vi "DragItem.vi"(8 "error in (no error)":errorcluster, 11 "OrderSelection in":refnum<class "OrderSelection.lvclass">) -> (0 "error out":errorcluster, 3 "OrderSelection out":refnum<class "OrderSelection.lvclass">)   [LabVIEW 2015, in "OrderSelection.lvclass"]
uses:
  OrderSelection.lvclass
  <vilib>/Utility/miscctls.llb/LVPointTypeDef.ctl
  OrderSelection.lvclass/OrderSelection.ctl
  Read ItemGraphic.vi
  Read Items.vi
  Read SelectedItem.vi
  <vilib>/Utility/inputDevices.llb/mouseAcquire.vi
  <vilib>/Utility/inputDevices.llb/closeMouse.vi
panel:
  out "SelectedItem":picture
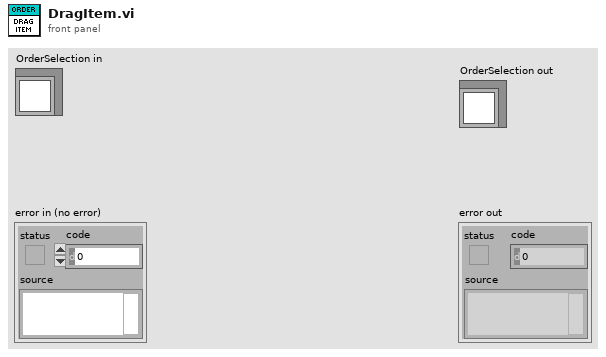
[diagram p1: front panel]
types:
  T1 = typedef "LVPointTypeDef.ctl" = cluster{"Horizontal":i16, "Vertical":i16}
  T2 = enum32{"Invalid", "Standard", "Closed", "Hidden", "Minimized", "Maximized"}
  T3 = cluster{"horizontal":enum16{"left", "center", "right"}, "vertical":enum16{"top", "center", "bottom"}}
  T4 = typedef "imagedata.ctl" = cluster{"image type":i32, "image depth":i32, "image":u8[], "mask":u8[], "colors":u32[], "Rectangle":cluster{"left":i16, "top":i16, "right":i16, "bottom":i16}}
  T5 = typedef "LVRectTypeDef.ctl" = cluster{"Left":i16, "Top":i16, "Right":i16, "Bottom":i16}
  T6 = cluster{"Horizontal":i32, "Vertical":i32, "Scrolling":i32}
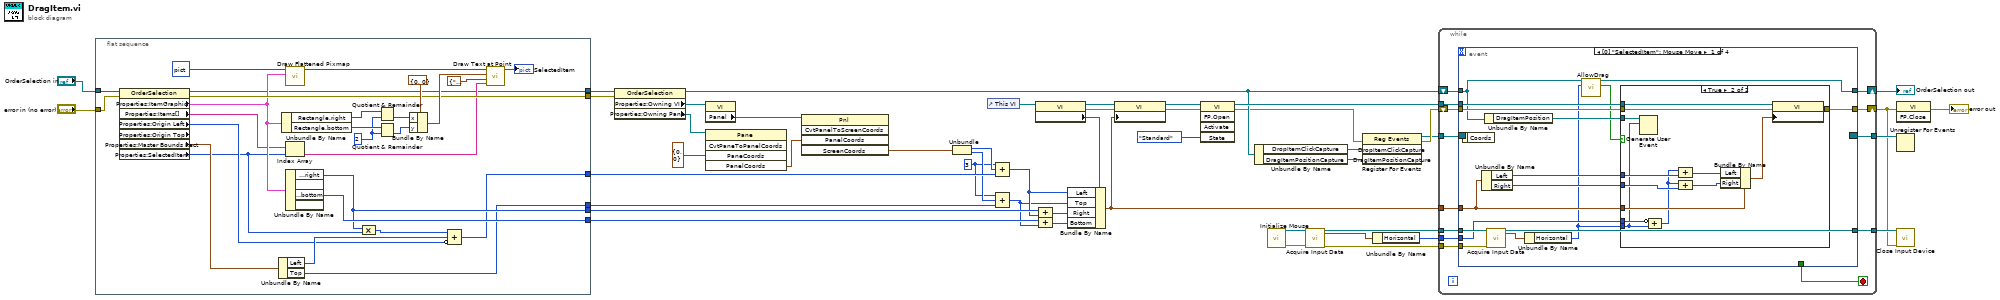
[diagram p0: block diagram]
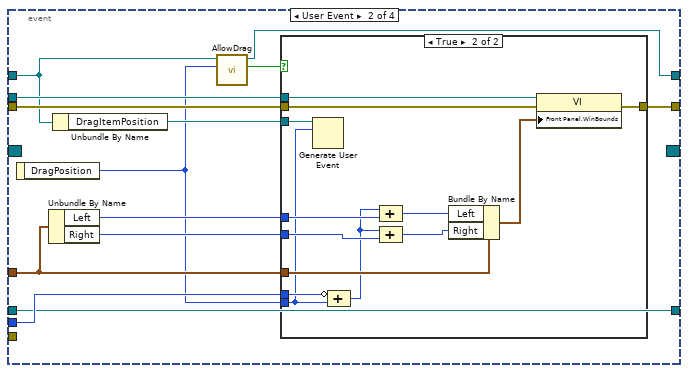
[diagram p3: hidden frame]
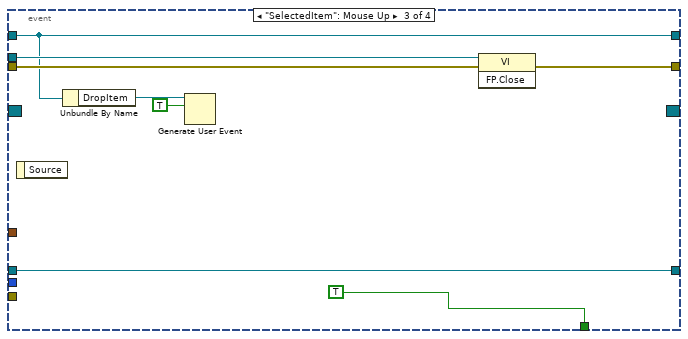
[diagram p5: hidden frame]
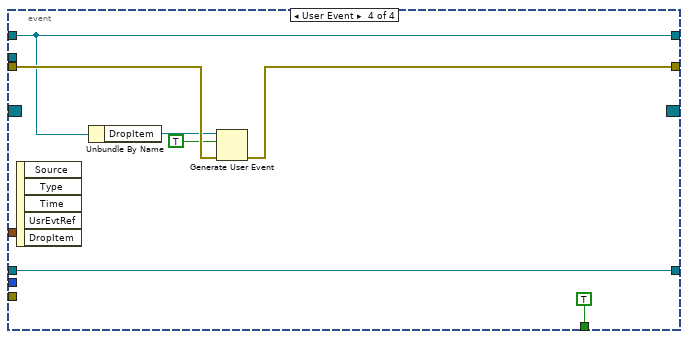
[diagram p6: hidden frame]
diagram:
  w26 = i16 3 ("value")
  n1 = flat-sequence {
    tunnel: "OrderSelection in" -> [w74]
    tunnel: "error in (no error)" -> [w62]
    tunnel: [w61] -> w45
    tunnel: [w55] -> w36
    tunnel: [w54] -> w35
    tunnel: [w51] -> w33
    tunnel: [w50] -> w28
    tunnel: [w49] -> w27
    frame #0 {
      w64 = i16 2 ("y")
      n2 = property class="OrderSelection" props=["Properties:ItemGraphic", "Properties:Items[]", "Properties:Origin Left", "Properties:Origin Top", "Properties:Master Bounds Rect", "Properties:SelectedItem"](reference=w74, error in=w62) -> (reference out=w50:refnum<class "OrderSelection.lvclass">, error out=w61:errorcluster, "Properties:ItemGraphic"=w60:T4, "Properties:Items[]"=w58:string[], "Properties:Origin Left"=w52:i16, "Properties:Master Bounds Rect"=w57:T5, "Properties:SelectedItem"=w48:i32)  [unwired: 1 out]
      n3 = Unbundle By Name(w57) -> ("Left"=w56:i16, "Top"=w49:i16)
      n4 = Unbundle By Name(w60) -> ("Rectangle.right"=w66:i16, "Rectangle.bottom"=w65:i16)
      n5 = call <vilib>:"Draw Flattened Pixmap.vi"("image data"=w60, "picture"=picture data[5B]) -> ("new picture"=w72:picture)  [unwired: 7 in]
      n6 = Index Array(array=w58, index=w48) -> (element=w59:string)
      n7 = Unbundle By Name(w60) -> ("Rectangle.right"=w54:i16, "Rectangle.bottom"=w55:i16)  [unwired: 2 out]
      n8 = Compound Arithmetic op=MULTIPLY(w54, w48) -> (w53:i32)
      n9 = Quotient & Remainder(x=w66, y=w64) -> (floor(x/y)=w67:i16)  [unwired: 1 out]
      n10 = Quotient & Remainder(x=w65, y=w64) -> (floor(x/y)=w63:i16)  [unwired: 1 out]
      n11 = Bundle By Name(cluster=cluster{"x":i16, "y":i16} {"x"=0, "y"=0} ("origin"), "x"=w67, "y"=w63) -> (w69:cluster{"x":i16, "y":i16})
      n12 = Compound Arithmetic op=ADD(w53, w56, invert w52) -> (w51:i32)
      n13 = call <vilib>:"Draw Text at Point.vi"("text"=w59, "alignment(left, top)"=T3 {"horizontal"=enum."center", "vertical"=enum."center"}, "origin"=w69, "picture"=w72) -> ("new picture"=→"SelectedItem":picture)  [unwired: 6 in, 1 out]
    }
  }
  n14 = property class="OrderSelection"(reference=w28, error in=w45) -> (reference out=w9:refnum<class "OrderSelection.lvclass">, "Properties:Owning VI"=w24:refnum<vi>, "Properties:Owning Pane"=w25:refnum<vi>)  [unwired: 1 out]
  n15 = property class="VI"(reference=w24) -> ("Panel"=w23:refnum<vi>)  [unwired: 1 in, 2 out]
  n16 = invoke class="Pane" method="CvtPaneToPanelCoords"(reference=w25, "PaneCoords"=T1 {"Horizontal"=0, "Vertical"=0} ("Panel Coordinates")) -> ("PanelCoords"=w22:T1)  [unwired: 3 in, 4 out]
  n17 = invoke class="Pnl" method="CvtPanelToScreenCoords"(reference=w23, "PanelCoords"=w22) -> ("ScreenCoords"=w21:T1)  [unwired: 3 in, 4 out]
  n18 = Unbundle(w21) -> ("Horizontal"=w31:i16, "Vertical"=w29:i16)
  n19 = control-ref of="This VI"() -> (w20:refnum<vi>)
  n20 = Compound Arithmetic op=ADD(w26, w31, w33) -> (w32:i32)
  n21 = Compound Arithmetic op=ADD(w26, w29, w27) -> (w30:i16)
  n22 = property class="VI"(reference=w20) -> (reference out=w42:refnum<vi>, error out=w43:errorcluster, "Front Panel.WinBounds"=w39:T5)  [unwired: 1 in]
  n23 = Compound Arithmetic op=ADD(w35, w32) -> (w38:i32)
  n24 = Compound Arithmetic op=ADD(w36, w30) -> (w37:i16)
  n25 = Bundle By Name(cluster=w39, "Left"=w32, "Top"=w30, "Right"=w38, "Bottom"=w37) -> (w18:T5)
  n26 = property class="VI"(reference=w42, error in=w43, "Front Panel.WinBounds"=w18) -> (reference out=w41:refnum<vi>, error out=w40:errorcluster)
  n27 = invoke class="VI" method="FP.Open"(reference=w41, error in=w40, "State"=T2."Standard") -> (reference out=w17:refnum<vi>, error out=w8:errorcluster)  [unwired: 2 in, 3 out]
  n28 = Unbundle By Name(w9) -> ("DropItemClickCapture"=w2:refnum<user-event>, "DragItemPositionCapture"=w1:refnum<user-event>)
  n29 = call <vilib>:"Initialize Mouse.vi"() -> ("error out"=w15:errorcluster, "device ID"=w16:refnum<k1>)  [unwired: 10 in]
  n30 = call-poly <vilib>:"Acquire Input Data.vi"("device ID"=w16, "error in (no error)"=w15) -> ("device ID"=w12:refnum<k1>, "axis info"=w14:T6, "error out"=w11:errorcluster)  [unwired: 14 in, 1 out]
  n31 = register-events(error in=w8, w2, w1) -> (reference out=w6:refnum<event-registration>, error out=w7:errorcluster)  [unwired: 1 in]
  n32 = Unbundle By Name(w14) -> ("Horizontal"=w13:i32)
  n33 = while {
    shift-right: [w87] -> w19
    shift-left: w9 -> [w86]
    shift-right: [w85] -> w3
    shift-left: w7 -> [w84]
    tunnel: w18 -> [w83]
    tunnel: w17 -> [w82]
    tunnel: w12 -> [w80]
    tunnel: w11 -> [w77]
    tunnel: [w79] -> w10
    tunnel: w13 -> [w78]
    tunnel: w6 -> [w76]
    tunnel: [w75] -> w5
    stop <- w81 stop-if-true
    n34 = event shown="[0] \"SelectedItem\": Mouse Move" {
      selector: w76 -> [_ _ _ _]
      dyn-events: [_ _ _ _] -> w75
      timeout: _ -> [_ _ _ _]
      tunnel: [w92 w123 w147 w155] -> w87
      tunnel: w86 -> [w93 w124 w147 w155]
      tunnel: [w98 w125 w150 w157] -> w85
      tunnel: w84 -> [w100 w127 w151 w158]
      tunnel: w83 -> [w102 w129 _ _]
      tunnel: w82 -> [w99 w126 w152 _]
      tunnel: [_ _ TRUE TRUE] -> w81
      tunnel: w80 -> [w97 w119 w148 w159]
      tunnel: [w95 w119 w148 w159] -> w79
      tunnel: w78 -> [w89 w120 _ _]
      tunnel: w77 -> [w96 _ _ _]
      event "SelectedItem": Mouse Move {
        n35 = event-data() -> ()  [unwired: 1 in, 1 out]
        n36 = Unbundle By Name(w102) -> ("Left"=w103:i16, "Right"=w101:i16)
        n37 = Unbundle By Name(w93) -> ("DragItemPosition"=w91:refnum<user-event>)
        n38 = call-poly <vilib>:"Acquire Input Data.vi"("device ID"=w97, "error in (no error)"=w96) -> ("device ID"=w95:refnum<k1>, "axis info"=w94:T6)  [unwired: 14 in, 2 out]
        n39 = Unbundle By Name(w94) -> ("Horizontal"=w88:i32)
        n40 = call "AllowDrag.vi"("DragPosition"=w88, "OrderSelection in"=w93) -> ("AllowDrag?"=w90:bool, "OrderSelection out"=w92:refnum<class "OrderSelection.lvclass">)  [unwired: 8 in]
        n41 = case shown="True" w90 {
          tunnel: w103 -> [_ w117]
          tunnel: w102 -> [_ w116]
          tunnel: w101 -> [_ w115]
          tunnel: w100 -> [w104 w112]
          tunnel: w99 -> [_ w111]
          tunnel: [w104 w110] -> w98
          tunnel: w89 -> [_ w108]
          tunnel: w91 -> [_ w106]
          tunnel: w88 -> [_ w105]
          frame False {
          }
          frame True {
            n42 = Generate User Event(user event=w106, event data cluster=w105) -> ()  [unwired: 2 in, 2 out]
            n43 = Compound Arithmetic op=ADD(invert w108, w105) -> (w107:i32)
            n44 = Compound Arithmetic op=ADD(w107, w117) -> (w114:i32)
            n45 = Compound Arithmetic op=ADD(w107, w115) -> (w113:i32)
            n46 = Bundle By Name(cluster=w116, "Left"=w114, "Right"=w113) -> (w109:T5)
            n47 = property class="VI"(reference=w111, error in=w112, "Front Panel.WinBounds"=w109) -> (error out=w110:errorcluster)  [unwired: 1 out]
          }
        }
      }
      event User Event {
        n48 = event-data() -> ("DragPosition"=w118:i32)  [unwired: 1 in]
        n49 = Unbundle By Name(w129) -> ("Left"=w130:i16, "Right"=w128:i16)
        n50 = Unbundle By Name(w124) -> ("DragItemPosition"=w122:refnum<user-event>)
        n51 = call "AllowDrag.vi"("DragPosition"=w118, "OrderSelection in"=w124) -> ("AllowDrag?"=w121:bool, "OrderSelection out"=w123:refnum<class "OrderSelection.lvclass">)  [unwired: 8 in]
        n52 = case shown="True" w121 {
          tunnel: w130 -> [_ w144]
          tunnel: w129 -> [_ w143]
          tunnel: w128 -> [_ w142]
          tunnel: w127 -> [w131 w139]
          tunnel: w126 -> [_ w138]
          tunnel: [w131 w137] -> w125
          tunnel: w120 -> [_ w135]
          tunnel: w122 -> [_ w133]
          tunnel: w118 -> [_ w132]
          frame False {
          }
          frame True {
            n53 = Generate User Event(user event=w133, event data cluster=w132) -> ()  [unwired: 2 in, 2 out]
            n54 = Compound Arithmetic op=ADD(invert w135, w132) -> (w134:i32)
            n55 = Compound Arithmetic op=ADD(w134, w144) -> (w141:i32)
            n56 = Compound Arithmetic op=ADD(w134, w142) -> (w140:i32)
            n57 = Bundle By Name(cluster=w143, "Left"=w141, "Right"=w140) -> (w136:T5)
            n58 = property class="VI"(reference=w138, error in=w139, "Front Panel.WinBounds"=w136) -> (error out=w137:errorcluster)  [unwired: 1 out]
          }
        }
      }
      event "SelectedItem": Mouse Up {
        n59 = event-data() -> ()  [unwired: 1 in, 1 out]
        n60 = Unbundle By Name(w147) -> ("DropItem"=w146:refnum<user-event>)
        n61 = Generate User Event(user event=w146, event data cluster=TRUE ("event data")) -> ()  [unwired: 2 in, 2 out]
        n62 = invoke class="VI" method="FP.Close"(reference=w152, error in=w151) -> (error out=w150:errorcluster)  [unwired: 1 in, 2 out]
      }
      event User Event {
        n63 = event-data() -> ()  [unwired: 1 in, 5 out]
        n64 = Unbundle By Name(w155) -> ("DropItem"=w154:refnum<user-event>)
        n65 = Generate User Event(user event=w154, event data cluster=TRUE ("event data"), error in=w158) -> (error out=w157:errorcluster)  [unwired: 1 in, 1 out]
      }
    }
  }
  "OrderSelection out" <- w19
  n66 = invoke class="VI" method="FP.Close"(error in=w3) -> (error out=→"error out":errorcluster)  [unwired: 2 in, 2 out]
  n67 = Unregister For Events(event registration refnum=w5) -> ()  [unwired: 1 in, 1 out]
  n68 = call-poly <vilib>:"Close Input Device.vi"("error in (no error)"=w3, "device ID"=w10) -> ()  [unwired: 8 in, 1 out]
